vi "Connect.vi"(8 "error in (no error)":errorcluster, 11 "MultiReader in":refnum<class "MultiReader.lvclass">) -> (0 "error out":errorcluster, 3 "MultiReader out":refnum<class "MultiReader.lvclass">)   [LabVIEW 2013, in "MultiReader.lvclass"]
doc: "Connect to the remote destination"
uses:
  MultiReader.lvclass
  BaseReader/BaseReader.lvclass
  MultiReader.lvclass/MultiReader.ctl
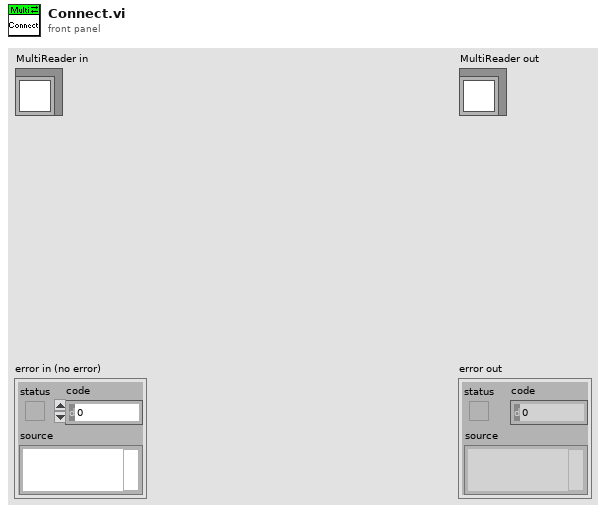
[diagram p1: front panel]
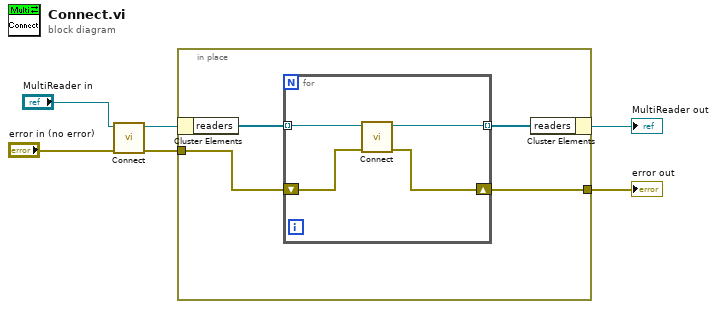
[diagram p0: block diagram]
diagram:
  n1 = call-parent "Connect.vi"("error in (no error)"="error in (no error)", "BaseReader in"="MultiReader in") -> ("error out"=w3:errorcluster, "BaseReader out"=w4:refnum<class "MultiReader.lvclass">)  [unwired: 8 in]
  n2 = in-place {
    in-place-border: [w8] -> w2
    in-place-border: w3 -> [w7]
    n3 = in-place-cluster #1(w4) -> ("readers"=w10:refnum<class "BaseReader.lvclass">[])
    n4 = for {
      tunnel: w10 -> [w14] mode=indexing
      tunnel: [w13] -> w9 mode=indexing
      shift-right: [w11] -> w8
      shift-left: w7 -> [w12]
      n5 = call-dynamic "Connect.vi"("error in (no error)"=w12, "BaseReader in"=w14) -> ("error out"=w11:errorcluster, "BaseReader out"=w13:refnum<class "BaseReader.lvclass">)  [unwired: 8 in]
    }
    n6 = in-place-cluster #1("readers"=w9) -> (→"MultiReader out":refnum<class "MultiReader.lvclass">)
  }
  "error out" <- w2
